vi "sendSyringeCommand.vi"(5 "Address":u16, 6 "Flow Direction (0: Dispense)":u16, 7 "Valve Position (1:Port A)":u16, 8 "error in (no error)":errorcluster, 9 "Number of Steps":u16, 11 "VISA Refnum in":refnum<visa-resource-name>) -> (0 "syringeError":errorcluster, 3 "VISA Refnum out":refnum<visa-resource-name>)   [LabVIEW 2021]
uses:
  globalVariables.vi
  Copy of Kloehn V6 Series Folder/Copy of Kloehn V6 Series.lvlib
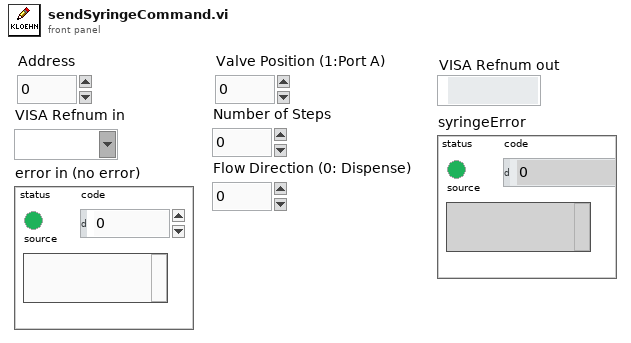
[diagram p1: front panel]
types:
  T1 = cluster{"Top Speed (5000 sps) ":i32, "Start Speed (750 sps)":i32, "Stop Speed (750 sps)":i32, "Accel (17500 st/s^2)":i32, "Decel (17500 st/s^2)":i32, "Backlash Steps (100 steps)":i32}
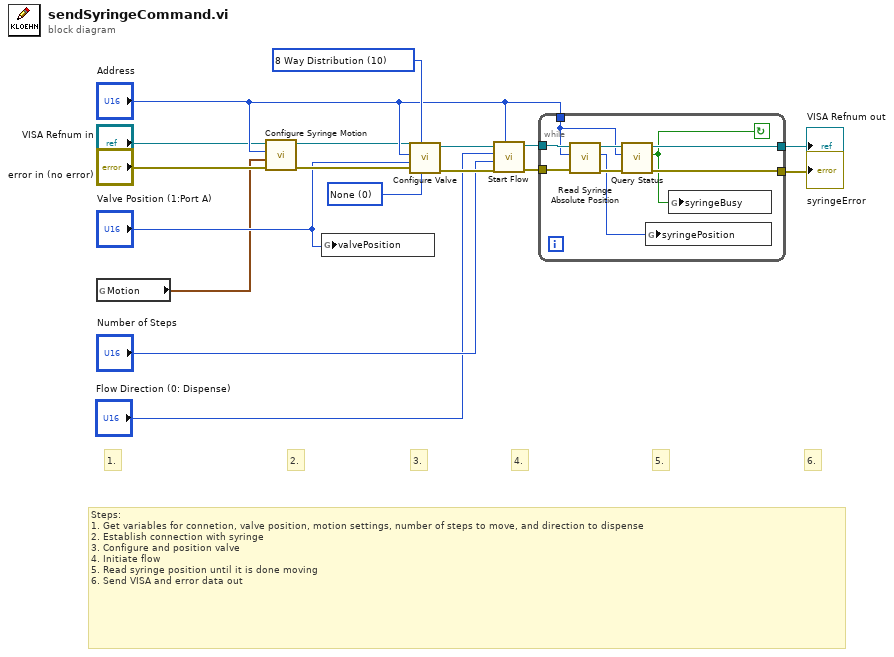
[diagram p0: block diagram]
diagram:
  w17 = u16 0 items=["None", "Bypass", "Input", "Output"] ("Three Way Valve Position (0:None)")
  w16 = u16 10 items=["None", "3 Way Non-Distribution", "3 Way Distribution", "4 Way Non-Distribution", "4 Way Distribution", "5 Way Non-Distribution", "5 Way Distribution", "6 Way Non-Distribution", "6 Way Distribution", "8 Way Non-Distribution", "8 Way Distribution", "12 Way Distribution", "2 Way Non-Distribution"] ("Valve Type (0:None)")
  # "Steps:\n1. Get variables for connetion, valve position, motion settings, number of steps to move, and direction to dispense\n2. Establish connection with syringe\n3. Configure and position valve\n4. Initiate flow\n5. Read syringe position until it is done moving\n6. Send VISA and error data out"
  # "6."
  # "5."
  # "3."
  # "2."
  # "1."
  # "4."
  n1 = global read "globalVariables.vi" "Motion"() -> (w1:T1)
  n2 = call "Configure Syringe Motion.vi"("error in (no error)"="error in (no error)", "Motion"=w1, "Address (1)"="Address", "VISA resource name"="VISA Refnum in") -> ("error out"=w13:errorcluster, "VISA resource name out"=w11:refnum<visa-resource-name>)  [unwired: 6 in]
  n3 = global write "globalVariables.vi" "valvePosition"("Valve Position (1:Port A)") -> ()
  n4 = call "Configure Valve.vi"("Three Way Valve Position (0:None)"=w17, "Valve Type (0:None)"=w16, "error in (no error)"=w13, "Valve Position (1:Port A)"="Valve Position (1:Port A)", "Address (1)"="Address", "VISA resource name"=w11) -> ("error out"=w14:errorcluster, "VISA resource name out"=w12:refnum<visa-resource-name>)  [unwired: 4 in]
  n5 = call "Start Flow.vi"("Address (1)"="Address", "error in (no error)"=w14, "Number of Steps (0)"="Number of Steps", "Flow Direction (0:Dispense)"="Flow Direction (0: Dispense)", "VISA resource name"=w12) -> ("error out"=w8:errorcluster, "VISA resource name out"=w7:refnum<visa-resource-name>)  [unwired: 4 in, 1 out]
  n6 = while {
    tunnel: w7 -> [w26]
    tunnel: w8 -> [w25]
    tunnel: [w22] -> w9
    tunnel: [w21] -> w10
    tunnel: "Address" -> [w20]
    stop <- w19 continue-if-true
    n7 = call "Read Syringe Absolute Position.vi"("error in (no error)"=w25, "Address (1)"=w20, "VISA resource name"=w26) -> ("error out"=w24:errorcluster, "Absolute Position"=w18:u16, "VISA resource name out"=w23:refnum<visa-resource-name>)  [unwired: 6 in]
    n8 = call "Query Status.vi"("error in (no error)"=w24, "Address (1)"=w20, "VISA resource name"=w23) -> ("error out"=w21:errorcluster, "Status"=w19:bool, "VISA resource name out"=w22:refnum<visa-resource-name>)  [unwired: 6 in]
    n9 = global write "globalVariables.vi" "syringePosition"(w18) -> ()
    n10 = global write "globalVariables.vi" "syringeBusy"(w19) -> ()
  }
  "syringeError" <- w10
  "VISA Refnum out" <- w9
